vi "Find Project Unit Tests.vi"(8 "error in (no error)":errorcluster {"code" format="Error %.0f"}, 10 "LabVIEW Project Path":path, 11 "DMC Test Runner in":refnum<class "DMC Test Runner.lvclass">) -> (0 "error out":errorcluster {"code" format="Error %.0f"}, 2 "Caraya Unit Tests":path[](array[path]), 3 "DMC Test Runner out":refnum<class "DMC Test Runner.lvclass">)   [LabVIEW 2023, in "DMC Test Runner.lvclass"]
doc: "Searches a LabVIEW project for all VIs and checks if a Caraya Unit Test should be run against it."
uses:
  DMC Test Runner.lvclass
  <vilib>/addons/_JKI Toolkits/Caraya/classes/Test Runner/Test Runner.lvclass
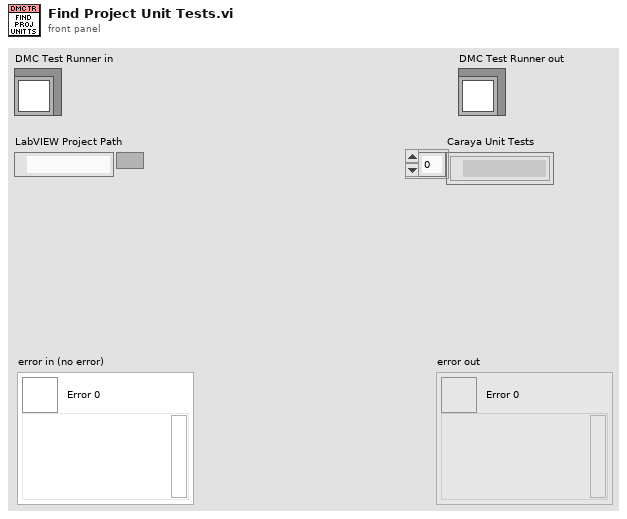
[diagram p1: front panel]
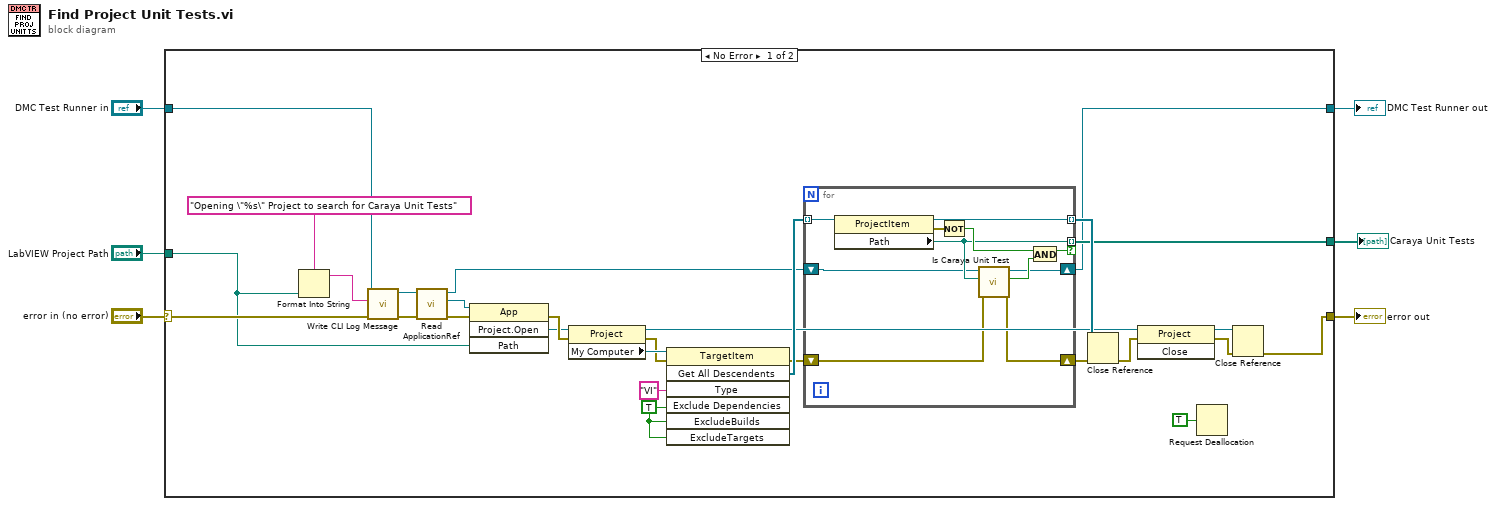
[diagram p0: block diagram]
diagram:
  n1 = case shown="No Error" "error in (no error)" {
    selector: "error in (no error)" -> [w34 w47]
    tunnel: [w19 w47] -> w5
    tunnel: [w10 w46] -> w3
    tunnel: "DMC Test Runner in" -> [w33 w46]
    tunnel: "LabVIEW Project Path" -> [w32 _]
    tunnel: [w18 _] -> w1
    frame No Error {
      w31 = TRUE ("ExcludeDependencies")
      n2 = Format Into String(format string="Opening \"%s\" Project to search for Caraya Unit Tests", w32) -> (resulting string=w16:string)  [unwired: 2 in, 1 out]
      n3 = call "Write CLI Log Message.vi"("error in (no error)"=w34, "Message"=w16, "DMC Test Runner in"=w33) -> ("error out"=w15:errorcluster, "DMC Test Runner out"=w12:refnum<class "DMC Test Runner.lvclass">)  [unwired: 7 in]
      n4 = call <vilib>:"Read ApplicationRef.vi"("error in (no error)"=w15, "Test Runner in"=w12) -> ("error out"=w14:errorcluster, "Application"=w13:refnum<vi>, "Test Runner out"=w11:refnum<class "DMC Test Runner.lvclass">)  [unwired: 7 in]
      n5 = invoke class="App" method="Project.Open"(reference=w13, error in=w14, "Path"=w32) -> (error out=w29:errorcluster, "Project:Open"=w24:refnum<vi>)  [unwired: 1 in, 2 out]
      n6 = property class="Project"(reference=w24, error in=w29) -> (reference out=w23:refnum<vi>, error out=w27:errorcluster, "My Computer"=w28:refnum<vi>)
      n7 = invoke class="TargetItem" method="Get All Descendents"(reference=w28, error in=w27, "Type"="VI", "Exclude Dependencies"=w31, "ExcludeBuilds"=w31, "ExcludeTargets"=w31) -> (error out=w9:errorcluster, "All Descendents"=w26:refnum<vi>[])  [unwired: 1 in, 5 out]
      n8 = for {
        tunnel: w26 -> [w45] mode=indexing
        tunnel: [w40] -> w18 mode=indexing if=w42
        tunnel: [w41] -> w25 mode=indexing
        shift-right: [w38] -> w10
        shift-left: w11 -> [w37]
        shift-right: [w35] -> w8
        shift-left: w9 -> [w36]
        n9 = property class="ProjectItem"(reference=w45) -> (reference out=w41:refnum<vi>, error out=w44:errorcluster, "Path"=w40:path)  [unwired: 1 in]
        n10 = Not(x=w44) -> (.not. x?=w43:bool)
        n11 = call "Is Caraya Unit Test.vi"("Error in"=w36, "VI Path"=w40, "DMC Test Runner in"=w37) -> ("Error out"=w35:errorcluster, "Contains Define Test.vi?"=w39:bool, "DMC Test Runner out"=w38:refnum<class "DMC Test Runner.lvclass">)  [unwired: 6 in]
        n12 = And(x=w43, y=w39) -> (x .and. y?=w42:bool)
      }
      n13 = Close Reference(reference=w25, error in (no error)=w8) -> (error out=w22:errorcluster)
      n14 = invoke class="Project" method="Close"(reference=w23, error in=w22) -> (reference out=w20:refnum<vi>, error out=w21:errorcluster)  [unwired: 1 in, 1 out]
      n15 = Request Deallocation(TRUE ("flag")) -> ()
      n16 = Close Reference(reference=w20, error in (no error)=w21) -> (error out=w19:errorcluster)
    }
    frame Error {
    }
  }
  "error out" <- w5
  "DMC Test Runner out" <- w3
  "Caraya Unit Tests" <- w1
